vi "draw a circle.vi"(5 "angular arc bounds":dbl=6.283185307179586, 6 "number of points":i32=20, 7 "angular arc center":dbl=3.141592653589793, 9 "center Y":dbl, 10 "center x":dbl, 11 "radius":dbl) -> (3 "output cluster":cluster{dbl[], dbl[]})   [LabVIEW 2018]
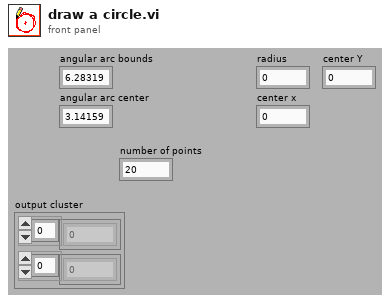
[diagram p1: front panel]
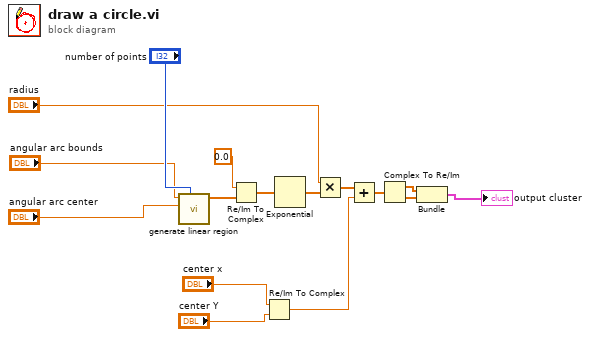
[diagram p0: block diagram]
diagram:
  n1 = call "generate linear region.vi"("number of  grid points"="number of points", "center"="angular arc center", "delta"="angular arc bounds") -> ("real axis"=w16:dbl[])  [unwired: 8 in]
  n2 = Re/Im To Complex(1:w16, 2:0.0) -> (0:w15:cdb[])
  n3 = Re/Im To Complex(1:"center Y", 2:"center x") -> (0:w1:cdb)
  n4 = Exponential(1:w15) -> (0:w14:cdb[])
  n5 = Multiply(x="radius", y=w14) -> (x*y=w13:cdb[])
  n6 = Add(x=w13, y=w1) -> (x+y=w12:cdb[])
  n7 = Complex To Re/Im(x + iy=w12) -> (x=w11:dbl[], y=w10:dbl[])
  n8 = Bundle(w11, w10) -> (→"output cluster":cluster{dbl[], dbl[]})  [unwired: 1 in]
